vi "Destroy Request Events.vi"(8 "error in":errorcluster) -> (0 "error out":errorcluster)   [LabVIEW 2024, in "UI Module Template.lvlib"]
doc: "Destroy the requests user events, even if there is an incoming error.\n\n<b>NOTE</b>: The contents of this VI are automatically generated and modified by the <b>Tools > DQMH Consortium > DQMH</b> utilities. Consider using those utilities instead of making your own modifications to this VI.\n_____\nBased on DQMH Project Template 7.0.1.1316."
uses:
  UI Module Template.lvlib
panel:
  # "NOTE: The contents of this VI are automatically generated and modified by the Tools > DQMH Consortium > DQMH utilities. Consider using those utilities instead of making your own modifications to this VI."
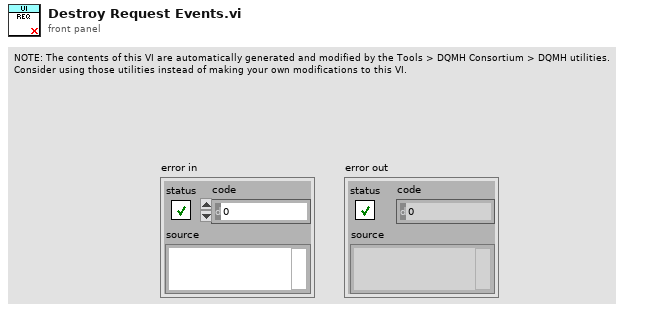
[diagram p1: front panel]
types:
  T1 = typedef "UI Module Template.lvlib/Request Events--cluster.ctl" = cluster{"Stop Module":refnum<user-event>, "Show Panel":refnum<user-event>, "Hide Panel":refnum<user-event>, "Get Module Execution Status":refnum<user-event>, "Show Diagram":refnum<user-event>, "Get UI Reference":refnum<user-event>, "Inserted Into Subpanel":refnum<user-event>, "Set Config (String)":refnum<user-event>, "Set Config":refnum<user-event>, "Get config":refnum<user-event>, "Get Config (String)":refnum<user-event>, "Private":cluster{"Generate Dummy Data":refnum<user-event>}}
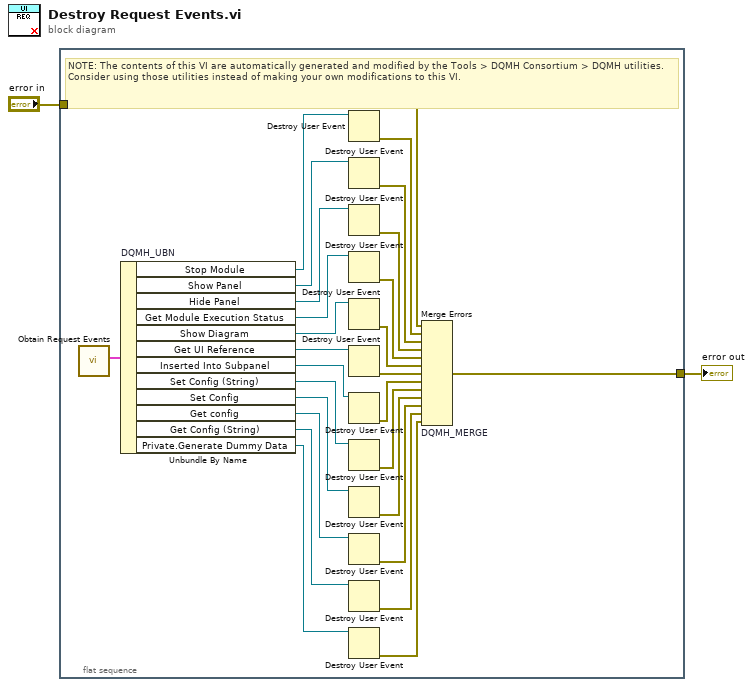
[diagram p0: block diagram]
diagram:
  n1 = flat-sequence {
    tunnel: [w28] -> w2
    tunnel: "error in" -> [w21]
    frame #0 {
      # "NOTE: The contents of this VI are automatically generated and modified by the Tools > DQMH Consortium > DQMH utilities. Consider using those utilities instead of making your own modifications to this VI."
      n2 = call "Obtain Request Events.vi"() -> ("UI Module Template Request Events"=w27:T1)  [unwired: 10 in, 1 out]
      n3 = Unbundle By Name "DQMH_UBN"(w27) -> ("Stop Module"=w26:refnum<user-event>, "Show Panel"=w23:refnum<user-event>, "Hide Panel"=w22:refnum<user-event>, "Get Module Execution Status"=w19:refnum<user-event>, "Show Diagram"=w17:refnum<user-event>, "Get UI Reference"=w15:refnum<user-event>, "Inserted Into Subpanel"=w13:refnum<user-event>, "Set Config (String)"=w11:refnum<user-event>, "Set Config"=w9:refnum<user-event>, "Get config"=w7:refnum<user-event>, "Get Config (String)"=w5:refnum<user-event>, "Private.Generate Dummy Data"=w3:refnum<user-event>)
      n4 = Destroy User Event(user event=w26) -> (error out=w29:errorcluster)  [unwired: 1 in]
      n5 = Destroy User Event(user event=w23) -> (error out=w25:errorcluster)  [unwired: 1 in]
      n6 = Destroy User Event(user event=w22) -> (error out=w24:errorcluster)  [unwired: 1 in]
      n7 = Destroy User Event(user event=w19) -> (error out=w20:errorcluster)  [unwired: 1 in]
      n8 = Destroy User Event(user event=w17) -> (error out=w18:errorcluster)  [unwired: 1 in]
      n9 = Destroy User Event(user event=w15) -> (error out=w16:errorcluster)  [unwired: 1 in]
      n10 = Destroy User Event(user event=w13) -> (error out=w14:errorcluster)  [unwired: 1 in]
      n11 = Destroy User Event(user event=w11) -> (error out=w12:errorcluster)  [unwired: 1 in]
      n12 = Destroy User Event(user event=w9) -> (error out=w10:errorcluster)  [unwired: 1 in]
      n13 = Destroy User Event(user event=w7) -> (error out=w8:errorcluster)  [unwired: 1 in]
      n14 = Destroy User Event(user event=w5) -> (error out=w6:errorcluster)  [unwired: 1 in]
      n15 = Destroy User Event(user event=w3) -> (error out=w4:errorcluster)  [unwired: 1 in]
      n16 = Merge Errors "DQMH_MERGE"(w21, w29, w25, w24, w20, w18, w16, w14, w12, w10, w8, w6, w4) -> (w28:errorcluster)
    }
  }
  "error out" <- w2
